vi "Accumulator.vi"(9 "Enable?":bool=TRUE, 10 "Reset?":bool, 11 "Value":dbl) -> (3 "Sum":dbl)   [LabVIEW 2019]
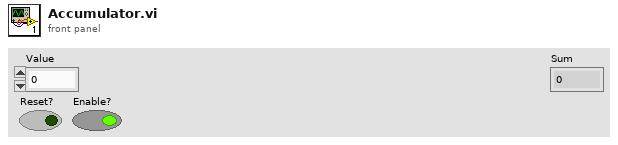
[diagram p1: front panel]
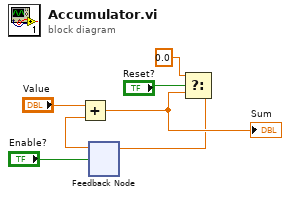
[diagram p0: block diagram]
diagram:
  n1 = feedback #1() -> (w7:dbl)  [unwired: 1 in]
  n2 = Add(x="Value", y=w7) -> (x+y=w3:dbl)
  "Sum" <- w3
  n3 = Select(t=0.0, s="Reset?", f=w3) -> (s? t:f=w2:dbl)
  n4 = feedback-in #1(w2, "Enable?") -> ()
